vi "Move.vi"(0 "X":dbl, 1 "Absolute":bool=TRUE, 5 "Y":dbl, 7 "Z":dbl, 9 "SpeedXY (mm/s)":dbl=100.0, 11 "SpeedZ (mm/s)":dbl=10.0, 12 "Move Z first":bool) -> (4 "Position Gcode":string)   [LabVIEW 2021]
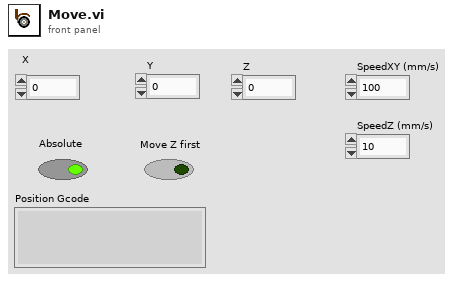
[diagram p1: front panel]
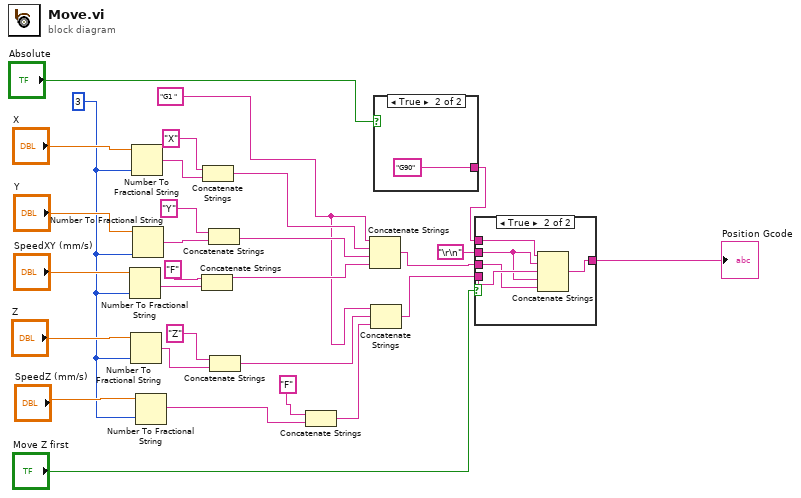
[diagram p0: block diagram]
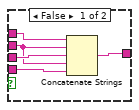
[diagram p2: hidden frame]
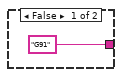
[diagram p3: hidden frame]
diagram:
  w9 = "G1 " ("string")
  w12 = 3
  n1 = Number To Fractional String(number="SpeedXY (mm/s)", precision (6)=w12) -> (F-format string=w17:string)  [unwired: 2 in]
  n2 = Number To Fractional String(number="Z", precision (6)=w12) -> (F-format string=w20:string)  [unwired: 2 in]
  n3 = Number To Fractional String(number="X", precision (6)=w12) -> (F-format string=w27:string)  [unwired: 2 in]
  n4 = Number To Fractional String(number="Y", precision (6)=w12) -> (F-format string=w25:string)  [unwired: 2 in]
  n5 = Number To Fractional String(number="SpeedZ (mm/s)", precision (6)=w12) -> (F-format string=w11:string)  [unwired: 2 in]
  n6 = Concatenate Strings("F", w17) -> (w15:string)
  n7 = Concatenate Strings("X", w27) -> (w23:string)
  n8 = Concatenate Strings("Y", w25) -> (w22:string)
  n9 = Concatenate Strings("Z", w20) -> (w8:string)
  n10 = Concatenate Strings("F", w11) -> (w7:string)
  n11 = Concatenate Strings(w9, w23, w22, w15) -> (w4:string)
  n12 = Concatenate Strings(w9, w8, w7) -> (w3:string)
  n13 = case shown="True" "Absolute" {
    tunnel: ["G91" "G90"] -> w6
    frame False {
    }
    frame True {
    }
  }
  n14 = case shown="True" "Move Z first" {
    tunnel: w6 -> [w36 w40]
    tunnel: "\r\n" -> [w34 w38]
    tunnel: w4 -> [w35 w37]
    tunnel: w3 -> [w33 w39]
    tunnel: [w32 w41] -> w1
    frame False {
      n15 = Concatenate Strings(w36, w34, w35, w34, w33) -> (w32:string)
    }
    frame True {
      n16 = Concatenate Strings(w40, w38, w39, w38, w37) -> (w41:string)
    }
  }
  "Position Gcode" <- w1
